vi "TcA02-002_ModifyingObjectsAttributesFromInheritedMethods.vi"(1 "Input buffer":T3="1", 3 "Invocation info":T2, 5 "error in (no error)":errorcluster, 6 "Add log to result?":bool) -> (16 "Test Data":T1 {"Numeric Measurement" format="%.2f"}, 19 "error out":errorcluster)   [LabVIEW 2009]
doc: "Test case template."
uses:
  Shared/Support_InputBuffer.ctl
  Shared/Support_InvocationInfo.ctl
  Shared/Support_TestData.ctl
  TestClasses/G#SubSubClass2_class/G#SubSubClass2.lvclass
  TestClasses/G#SubClass2_class/G#SubClass2.lvclass
  TestClasses/G#BaseClass2_class/G#BaseClass2.lvclass
  <vilib>/addons/_AddQ/G#Object/G#Object.lvclass
panel:
  in  "Test name":string="TcA02-002 Modifying objects attributes from inherited methods"
  out "Test result":bool
  out "Result":string
  # "Verify that an object can read and set the attributes\nfrom methods inherited from base classes."
  # "Sub test case"
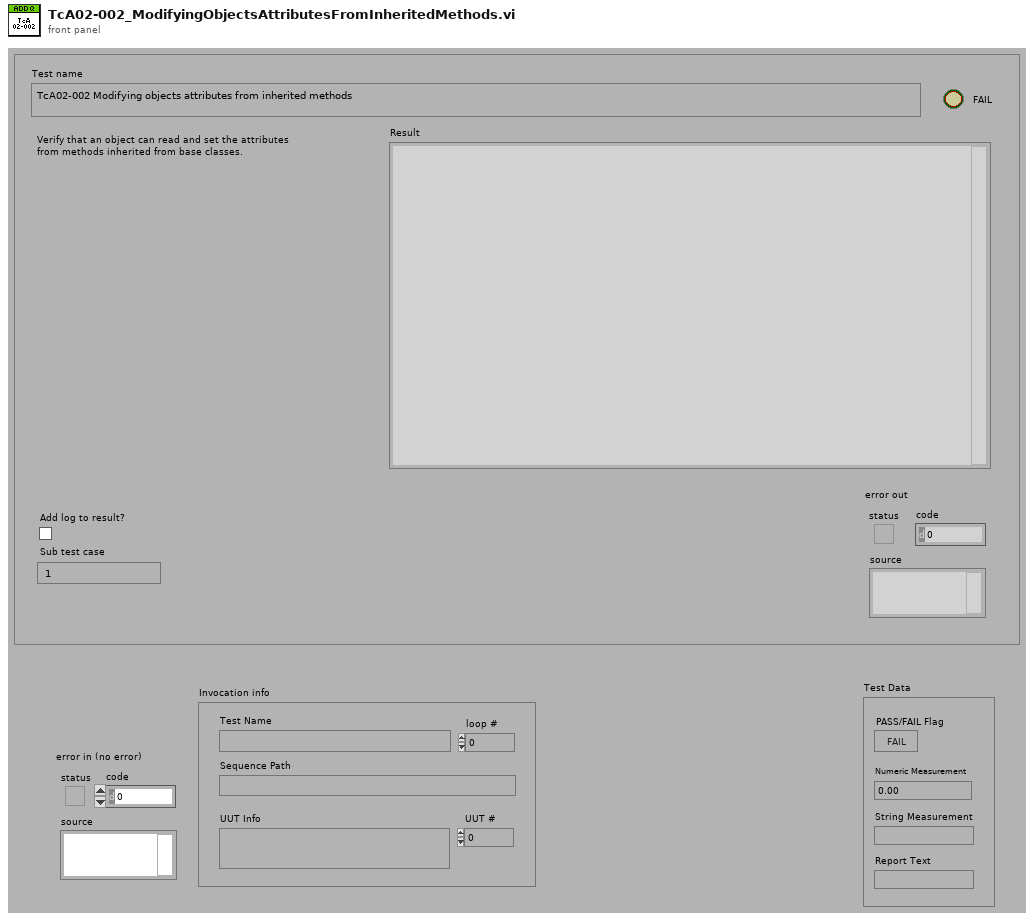
[diagram p1: front panel]
types:
  T1 = typedef "Support_TestData.ctl" = cluster{"PASS/FAIL Flag":bool, "Numeric Measurement":dbl, "String Measurement":string, "Report Text":string}
  T2 = typedef "Support_InvocationInfo.ctl" = cluster{"UUT #":i32, "loop #":i32, "UUT Info":string, "Test Name":string, "Sequence Path":path}
  T3 = typedef "Support_InputBuffer.ctl" = string
  T4 = typedef "Support_ResultType.ctl" = cluster{"Pass":bool, "Comment":string, "MeasurementValue":dbl}
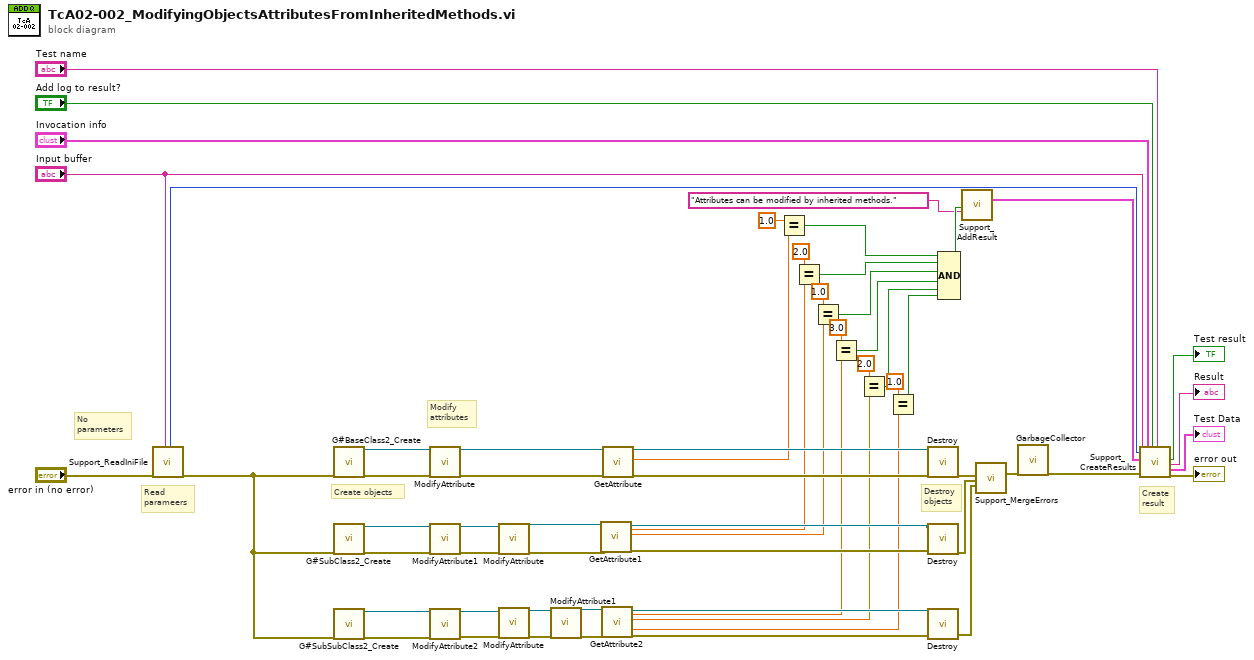
[diagram p0: block diagram]
diagram:
  # "Destroy\nobjects"
  # "Create objects"
  # "Modify\nattributes"
  # "No\nparameters"
  # "Create\nresult"
  # "Read\nparameers"
  n1 = call "Support_ReadIniFile.vi"("error in (no error)"="error in (no error)", "Sub test case"="Input buffer") -> ("Timer start"=w52:u32, "error out"=w51:errorcluster)  [unwired: 10 in, 6 out]
  n2 = call "G#BaseClass2_Create.vi"("error in (no error)"=w51) -> ("reference out"=w17:refnum<class "G#BaseClass2.lvclass">, "error out"=w14:errorcluster)  [unwired: 17 in]
  n3 = call "G#SubClass2_Create.vi"("error in (no error)"=w51) -> ("reference out"=w18:refnum<class "G#SubClass2.lvclass">, "error out"=w15:errorcluster)  [unwired: 17 in]
  n4 = call "G#SubSubClass2_Create.vi"("error in (no error)"=w51) -> ("reference out"=w19:refnum<class "G#SubSubClass2.lvclass">, "error out"=w16:errorcluster)  [unwired: 17 in]
  n5 = call-dynamic "ModifyAttribute.vi"("reference in"=w17, "error in (no error)"=w14) -> ("reference out"=w42:refnum<class "G#BaseClass2.lvclass">, "error out"=w13:errorcluster)  [unwired: 15 in, 1 out]
  n6 = call-dynamic "ModifyAttribute1.vi"("reference in"=w18, "error in (no error)"=w15) -> ("reference out"=w12:refnum<class "G#SubClass2.lvclass">, "error out"=w11:errorcluster)  [unwired: 15 in, 1 out]
  n7 = call-dynamic "ModifyAttribute2.vi"("reference in"=w19, "error in (no error)"=w16) -> ("reference out"=w7:refnum<class "G#SubSubClass2.lvclass">, "error out"=w8:errorcluster)  [unwired: 15 in, 1 out]
  n8 = call-dynamic "ModifyAttribute.vi"("reference in"=w12, "error in (no error)"=w11) -> ("reference out"=w9:refnum<class "G#SubClass2.lvclass">, "error out"=w10:errorcluster)  [unwired: 15 in, 1 out]
  n9 = call-dynamic "ModifyAttribute.vi"("reference in"=w7, "error in (no error)"=w8) -> ("reference out"=w6:refnum<class "G#SubSubClass2.lvclass">, "error out"=w5:errorcluster)  [unwired: 15 in, 1 out]
  n10 = call-dynamic "ModifyAttribute1.vi"("reference in"=w6, "error in (no error)"=w5) -> ("reference out"=w3:refnum<class "G#SubSubClass2.lvclass">, "error out"=w4:errorcluster)  [unwired: 15 in, 1 out]
  n11 = call-dynamic "GetAttribute1.vi"("reference in"=w9, "error in (no error)"=w10) -> ("reference out"=w40:refnum<class "G#SubClass2.lvclass">, "Base class.Numeric"=w35:dbl, "SubAttribute"=w33:dbl, "error out"=w43:errorcluster)  [unwired: 12 in, 2 out]
  n12 = call-dynamic "GetAttribute2.vi"("reference in"=w3, "error in (no error)"=w4) -> ("reference out"=w39:refnum<class "G#SubSubClass2.lvclass">, "Base class.Base class.Numeric"=w31:dbl, "Base class.SubAttribute"=w28:dbl, "SubSubAttribute"=w27:dbl, "error out"=w44:errorcluster)  [unwired: 11 in, 2 out]
  n13 = call-dynamic "GetAttribute.vi"("reference in"=w42, "error in (no error)"=w13) -> ("reference out"=w41:refnum<class "G#BaseClass2.lvclass">, "Numeric"=w38:dbl, "error out"=w45:errorcluster)  [unwired: 13 in, 2 out]
  n14 = Equal?(x=1.0, y=w38) -> (x = y?=w26:bool)
  n15 = Equal?(x=2.0, y=w35) -> (x = y?=w25:bool)
  n16 = Equal?(x=1.0, y=w33) -> (x = y?=w24:bool)
  n17 = Equal?(x=3.0, y=w31) -> (x = y?=w23:bool)
  n18 = Equal?(x=2.0, y=w28) -> (x = y?=w22:bool)
  n19 = Equal?(x=1.0, y=w27) -> (x = y?=w21:bool)
  n20 = call-dynamic "Destroy.vi"("reference in"=w41, "error in (no error)"=w45) -> ("error out"=w50:errorcluster)  [unwired: 16 in, 1 out]
  n21 = call-dynamic "Destroy.vi"("reference in"=w40, "error in (no error)"=w43) -> ("error out"=w49:errorcluster)  [unwired: 16 in, 1 out]
  n22 = call-dynamic "Destroy.vi"("reference in"=w39, "error in (no error)"=w44) -> ("error out"=w48:errorcluster)  [unwired: 16 in, 1 out]
  n23 = Compound Arithmetic op=AND(w26, w25, w24, w23, w22, w21) -> (w20:bool)
  n24 = call "Support_AddResult.vi"("Pass"=w20, "Comment"="Attributes can be modified by inherited methods.") -> ("Results out"=w2:T4[])  [unwired: 17 in]
  n25 = call "Support_MergeErrors.vi"("error in 1"=w50, "error in 2"=w49, "error in 3"=w48) -> ("error out"=w47:errorcluster)  [unwired: 15 in, 1 out]
  n26 = call <vilib>:"GarbageCollector.vi"("error in (no error)"=w47) -> ("error out"=w46:errorcluster)  [unwired: 16 in, 2 out]
  n27 = call "Support_CreateResults.vi"("Sub test case"="Input buffer", "Timer start"=w52, "Results"=w2, "error in (no error)"=w46, "Invocation info"="Invocation info", "Add log to result?"="Add log to result?", "Test name"="Test name") -> ("Pass/fail flag"=→"Test result":bool, "Result"=→"Result":string, "Test Data"=→"Test Data":T1, "error out"=→"error out":errorcluster)  [unwired: 9 in]
